vi "main.vi"() -> ()   [LabVIEW 2020]
panel:
  out "x+y":dbl
  in  "y":dbl
  in  "x":dbl
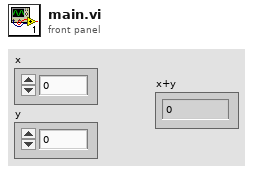
[diagram p1: front panel]
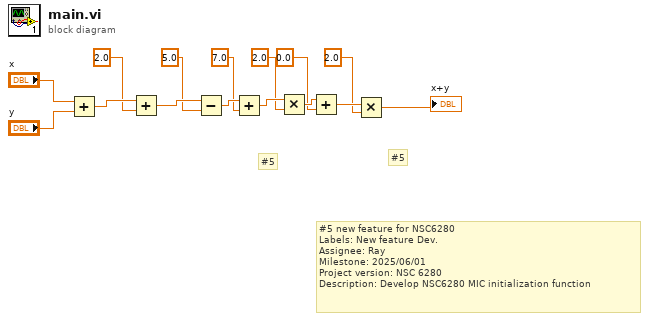
[diagram p0: block diagram]
diagram:
  # "#5"
  # "#5"
  # "#5 new feature for NSC6280 \nLabels: New feature Dev.\nAssignee: Ray\nMilestone: 2025/06/01\nProject version: NSC 6280\nDescription: Develop NSC6280 MIC initialization function"
  n1 = Add(x="x", y="y") -> (x+y=w13:dbl)
  n2 = Add(x=w13, y=2.0) -> (x+y=w11:dbl)
  n3 = Subtract(x=w11, y=5.0) -> (x-y=w9:dbl)
  n4 = Add(x=w9, y=7.0) -> (x+y=w7:dbl)
  n5 = Multiply(x=w7, y=2.0) -> (x*y=w5:dbl)
  n6 = Add(x=w5, y=0.0) -> (x+y=w3:dbl)
  n7 = Multiply(x=w3, y=2.0) -> (x*y=→"x+y":dbl)
